vi "Init.vi"(8 "error in (no error)":errorcluster, 9 "Computer Specifier":u8, 11 "Channel Manager in":refnum<class "Channel Manager.lvclass">) -> (0 "error out":errorcluster, 3 "Channel Manager out":refnum<class "Channel Manager.lvclass">)   [LabVIEW 2018, in "Channel Manager.lvclass"]
uses:
  Channel Manager.lvclass
  Channel/Channel.lvclass
  Channel/Channel.lvclass/Channel.ctl
  Channel Manager.lvclass/Channel Manager.ctl
panel:
  in  "Channel.lvclass":refnum<class "Channel.lvclass">
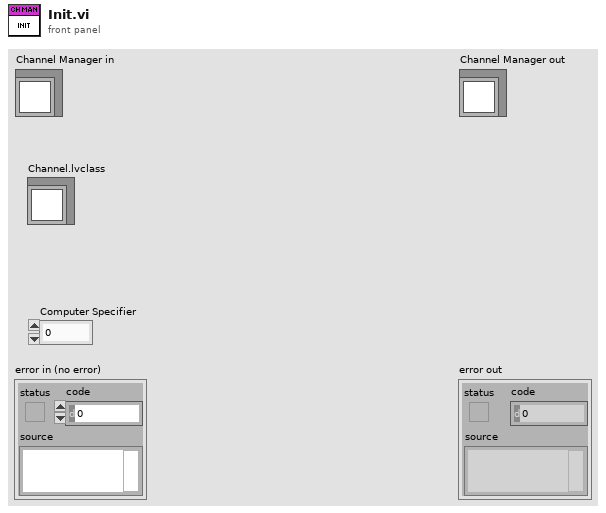
[diagram p1: front panel]
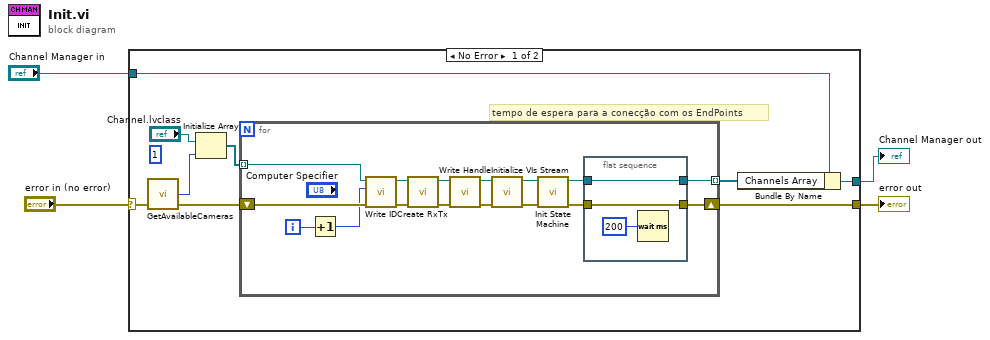
[diagram p0: block diagram]
diagram:
  n1 = case shown="No Error" "error in (no error)" {
    selector: "error in (no error)" -> [w6 w34]
    tunnel: [w13 w34] -> w3
    tunnel: [w7 w33] -> w1
    tunnel: "Channel Manager in" -> [w8 w33]
    frame No Error {
      (unwired) 1
      # "tempo de espera para a conecção com os EndPoints"
      n2 = call <userlib>:"GetAvailableCameras.vi"("error in (no error)"=w6) -> ("error out"=w11:errorcluster, "totalCameras"=w5:i32)  [unwired: 2 in, 1 out]
      n3 = Initialize Array("Channel.lvclass", w5) -> (w9:refnum<class "Channel.lvclass">[])
      n4 = for {
        tunnel: [w18] -> w12 mode=indexing
        shift-right: [w16] -> w13
        shift-left: w11 -> [w29]
        tunnel: w9 -> [w28] mode=indexing
        i -> [w15]
        n5 = Increment(x=w15) -> (x+1=w14:i32)
        n6 = call "Write ID.vi"("error in (no error)"=w29, "ID"=w14, "Channel in"=w28) -> ("error out"=w24:errorcluster, "Channel out"=w27:refnum<class "Channel.lvclass">)  [unwired: 7 in]
        n7 = call "Create RxTx.vi"("error in (no error)"=w24, "Channel in"=w27) -> ("error out"=w25:errorcluster, "Channel out"=w26:refnum<class "Channel.lvclass">)  [unwired: 8 in]
        n8 = call "Write Handle.vi"("error in (no error)"=w25, "Channel in"=w26) -> ("error out"=w22:errorcluster, "Channel out"=w23:refnum<class "Channel.lvclass">)  [unwired: 8 in]
        n9 = call "Initialize VIs Stream.vi"("error in (no error)"=w22, "Channel in"=w23) -> ("error out"=w20:errorcluster, "Channel out"=w21:refnum<class "Channel.lvclass">)  [unwired: 8 in]
        n10 = call "Init State Machine.vi"("error in (no error)"=w20, "Channel in"=w21) -> ("error out"=w17:errorcluster, "Channel out"=w19:refnum<class "Channel.lvclass">)  [unwired: 8 in]
        n11 = flat-sequence {
          tunnel: w19 -> [w32]
          tunnel: [w32] -> w18
          tunnel: w17 -> [w31]
          tunnel: [w31] -> w16
          frame #0 {
            n12 = Wait (ms)(milliseconds to wait=u32 200) -> ()  [unwired: 1 out]
          }
        }
      }
      n13 = Bundle By Name(cluster=w8, "Channels Array"=w12) -> (w7:refnum<class "Channel Manager.lvclass">)
    }
    frame Error {
    }
  }
  "error out" <- w3
  "Channel Manager out" <- w1
